vi "GOOP_ProviderName_Translator.vi"(11 "AllClassProvidersIn":string[](array[string])) -> (3 "ClassProvidersTranslatedNamesOut":string[](array[string]))   [LabVIEW 2020]
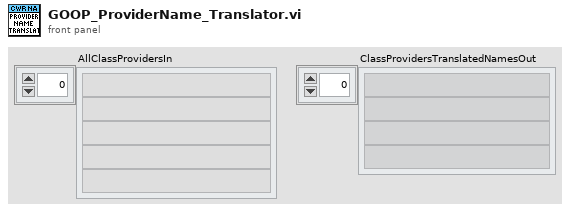
[diagram p1: front panel]
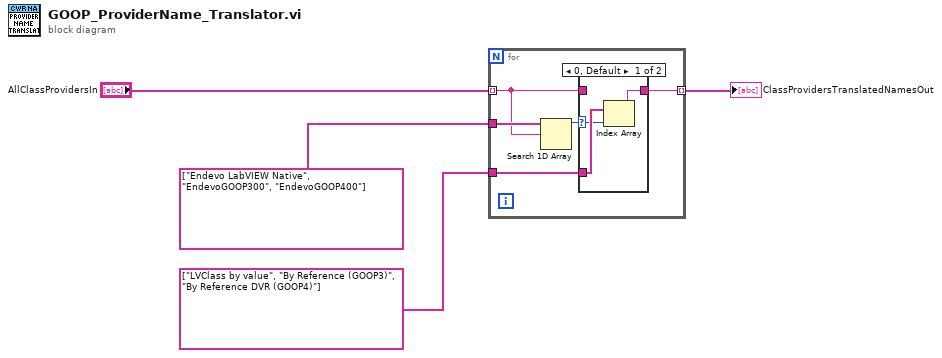
[diagram p0: block diagram]
diagram:
  n1 = for {
    tunnel: [w6] -> w4 mode=indexing
    tunnel: "AllClassProvidersIn" -> [w7] mode=indexing
    tunnel: string[] ["Endevo LabVIEW Native", "EndevoGOOP300", "EndevoGOOP400"] ("AllClassProviders") -> [w9]
    tunnel: string[] ["LVClass by value", "By Reference (GOOP3)", "By Reference DVR (GOOP4)"] ("AllClassProviders") -> [w5]
    n2 = Search 1D Array(1D array=w9, element=w7) -> (index of element=w8:i32)  [unwired: 1 in]
    n3 = case shown="0, Default" w8 {
      selector: w8 -> [w11 _]
      tunnel: w7 -> [_ w13]
      tunnel: [w10 w13] -> w6
      tunnel: w5 -> [w12 _]
      frame 0, Default {
        n4 = Index Array(array=w12, index=w11) -> (element=w10:string)
      }
      frame -1 {
      }
    }
  }
  "ClassProvidersTranslatedNamesOut" <- w4
